vi "Chroma 1905x Series Configure IR RANGE AUTO Query.vi"(8 "error in (no error)":errorcluster, 10 "Step":T1=1 min=1 max=99 step=1, 11 "VISA resource name":refnum<visa-resource-name>) -> (0 "error out":errorcluster, 2 "Result":string, 3 "VISA resource name out":refnum<visa-resource-name>)   [LabVIEW 2025]
uses:
  Type Def/steps--numeric.ctl
panel:
  # "RANGE AUTO query"
  # "(for IR mode ONLY)"
  # "0=Off /1=On"
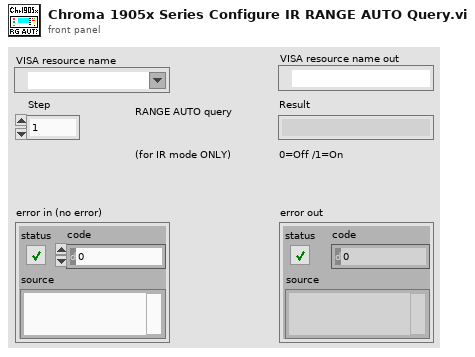
[diagram p1: front panel]
types:
  T1 = typedef "steps--numeric.ctl" = u8
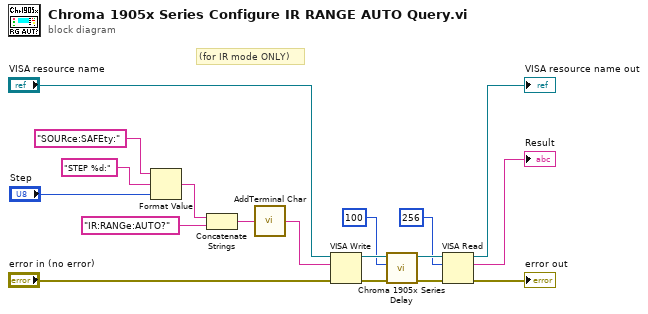
[diagram p0: block diagram]
diagram:
  # "(for IR mode ONLY)"
  n1 = Format Value(string ("")="SOURce:SAFEty:", format string="STEP %d:", value (0)="Step") -> (output string=w15:string)
  n2 = Concatenate Strings(w15, "IR:RANGe:AUTO?") -> (w13:string)
  n3 = call "AddTerminal Char.vi"("Cmd string"=w13) -> ("Concatenated String"=w5:string)  [unwired: 4 in]
  n4 = VISA Write(VISA resource name="VISA resource name", write buffer=w5, error in (no error)="error in (no error)") -> (VISA resource name out=w10:refnum<visa-resource-name>, error out=w12:errorcluster)  [unwired: 1 out]
  n5 = call "Chroma 1905x Series Delay.vi"("error in (no error)"=w12, "Time Delay [ms]"=u32 100 ("Time Delay ms"), "VISA resource name"=w10) -> ("error out"=w11:errorcluster, "VISA resource name 2"=w9:refnum<visa-resource-name>)  [unwired: 7 in]
  n6 = VISA Read(VISA resource name=w9, byte count=u32 256, error in (no error)=w11) -> (VISA resource name out=→"VISA resource name out":refnum<visa-resource-name>, read buffer=→"Result":string, error out=→"error out":errorcluster)  [unwired: 1 out]
